vi "Stage 3.4 Placing hardware into subVIs.vi"() -> ()   [LabVIEW 2020]
uses:
  HRM-Stage3-User_events.ctl
  HRM-Stage3-init_cluster.ctl
panel:
  out "Process Error":errorcluster
  out "error out":errorcluster
  out "error out Hardware":errorcluster
  in  "Addition signal to remove (0) [s]":dbl
  out "Pulse":dbl
  out "Filtered":waveform(dbl)(graph)
  in  "Samples size (10) [s]":i32=10
  out "unfiltered wf":waveform(dbl)(graph)
  in  "Stop":bool
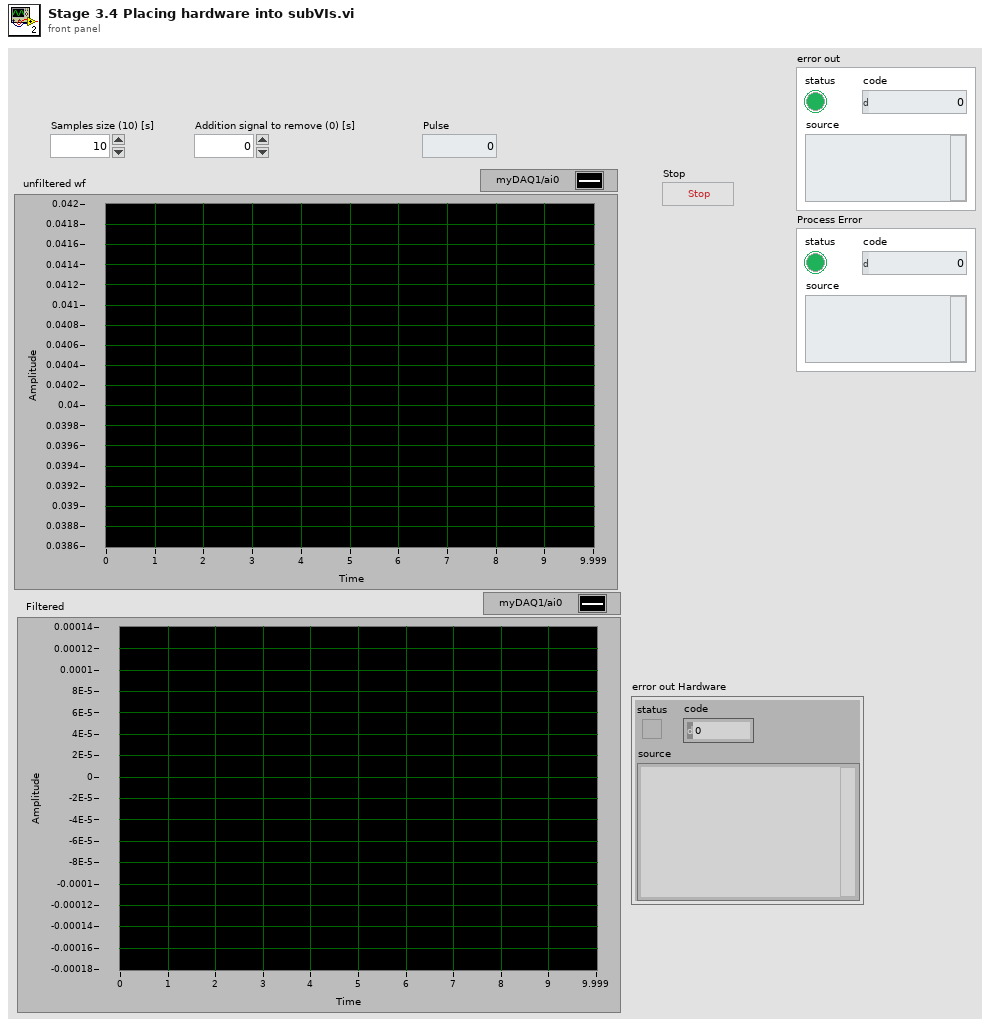
[diagram p1: front panel]
types:
  T1 = typedef "HRM-Stage3-init_cluster.ctl" = cluster{"User events":T2}
  T2 = typedef "HRM-Stage3-User_events.ctl" = cluster{"Signal to remove":refnum<user-event>, "Sample size":refnum<user-event>, "Filtered wf":refnum<user-event>, "Unfiltered wf":refnum<user-event>, "Raw wf":refnum<user-event>, "Pulse":refnum<user-event>, "Stop":refnum<user-event>, "Feedback":refnum<user-event>}
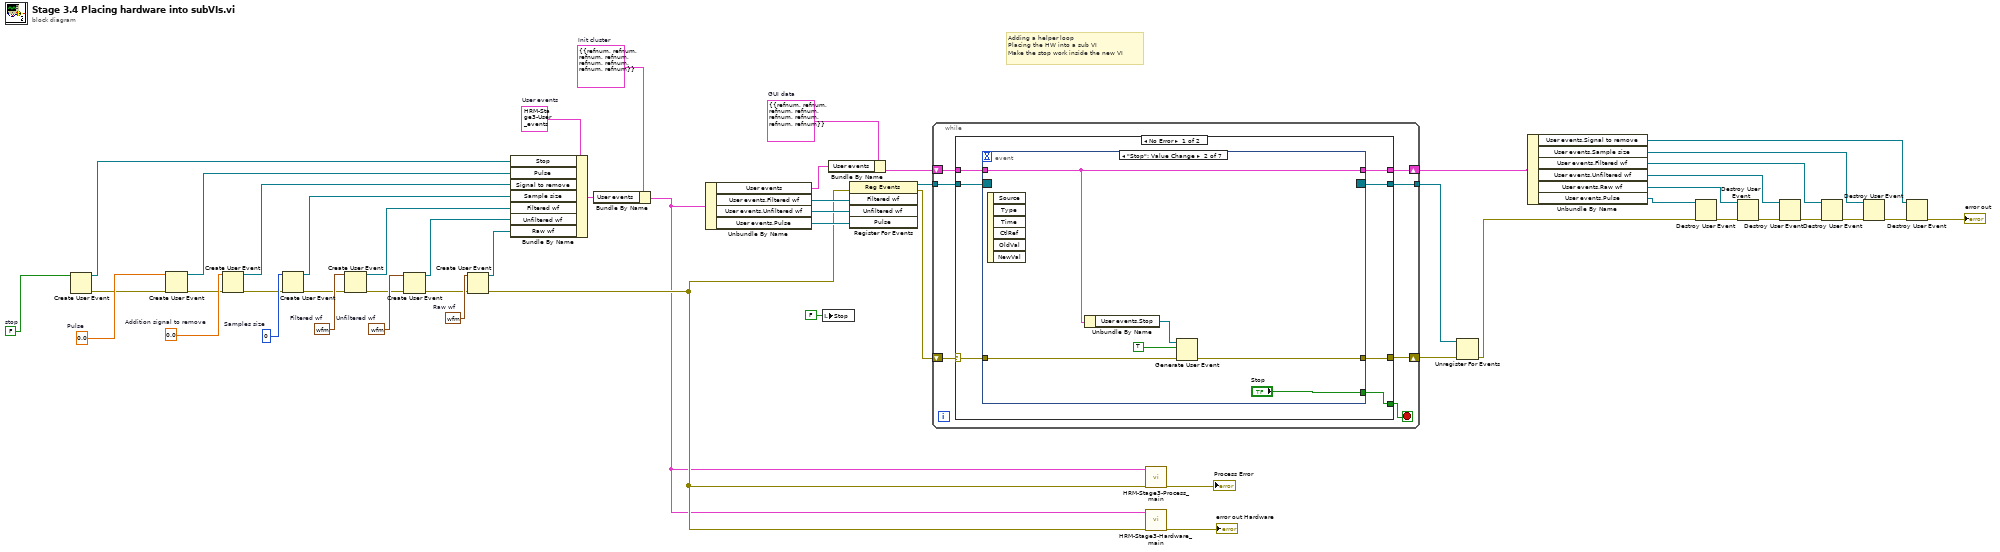
[diagram p0: block diagram]
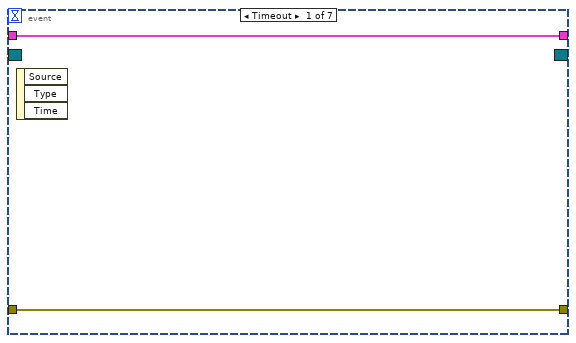
[diagram p2: hidden frame]
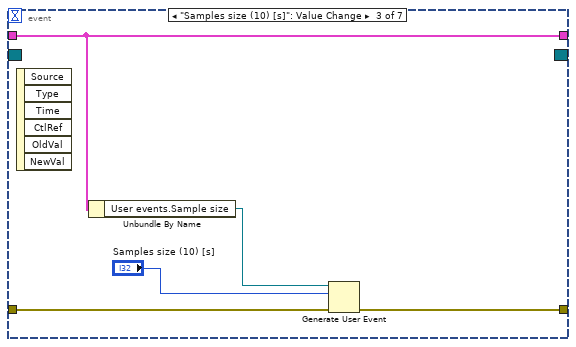
[diagram p3: hidden frame]
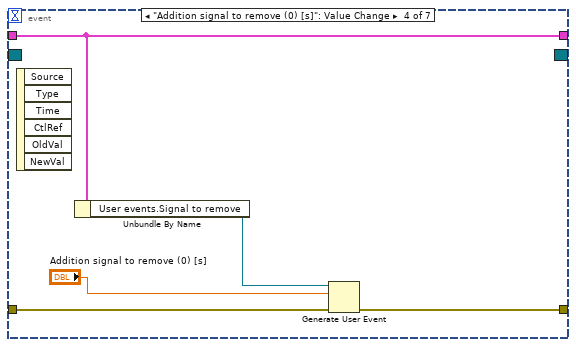
[diagram p4: hidden frame]
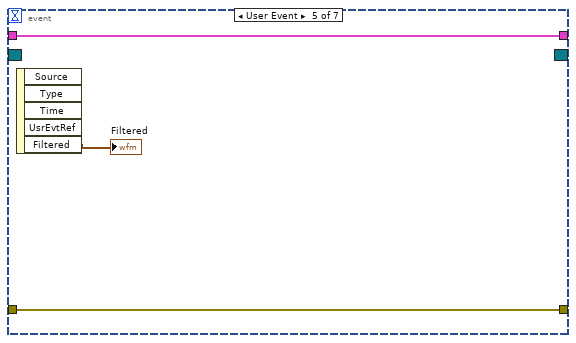
[diagram p5: hidden frame]
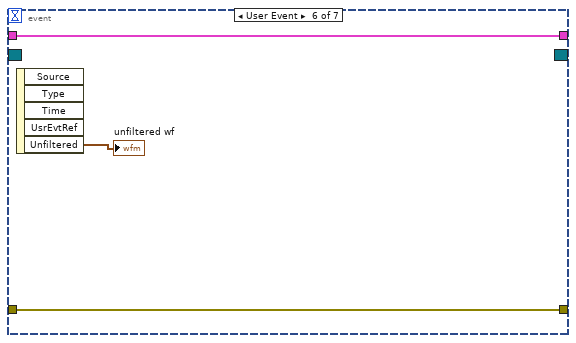
[diagram p6: hidden frame]
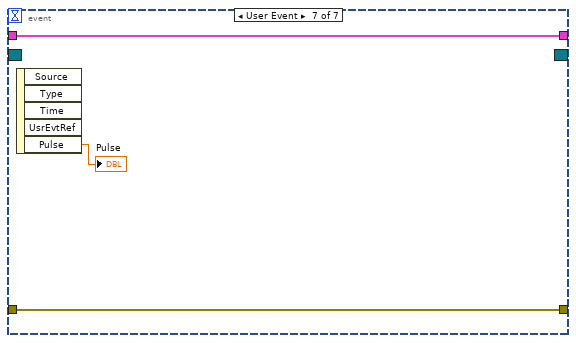
[diagram p7: hidden frame]
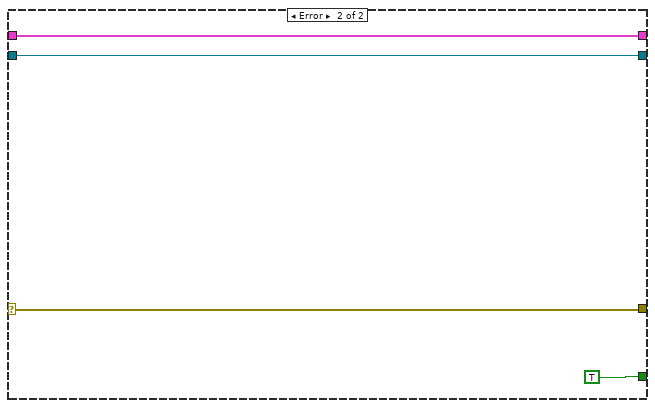
[diagram p8: hidden frame]
diagram:
  w8 = FALSE  # stop
  w14 = T1 {"User events"={"Signal to remove"=refnum, "Sample size"=refnum, "Filtered wf"=refnum, "Unfiltered wf"=refnum, "Raw wf"=refnum, "Pulse"=refnum, "Stop"=refnum, "Feedback"=refnum}}  # Init cluster
  w33 = cluster{"User events":T2} {"User events"={"Signal to remove"=refnum, "Sample size"=refnum, "Filtered wf"=refnum, "Unfiltered wf"=refnum, "Raw wf"=refnum, "Pulse"=refnum, "Stop"=refnum, "Feedback"=refnum}}  # GUI data
  w37 = 0.0  # Pulse
  w43 = T2 {"Signal to remove"=refnum, "Sample size"=refnum, "Filtered wf"=refnum, "Unfiltered wf"=refnum, "Raw wf"=refnum, "Pulse"=refnum, "Stop"=refnum, "Feedback"=refnum}  # User events
  w48 = 0  # Samples size
  w49 = 0.0  # Addition signal to remove
  w50 = waveform(dbl) {"t0"=timestamp(0 s since 1904-01-01), "dt"=1.0, "Y"=[]}  # Filtered wf
  w51 = waveform(dbl) {"t0"=timestamp(0 s since 1904-01-01), "dt"=1.0, "Y"=[]}  # Unfiltered wf
  w52 = waveform(dbl) {"t0"=timestamp(0 s since 1904-01-01), "dt"=1.0, "Y"=[]}  # Raw wf
  # "Adding a helper loop\nPlacing the HW into a sub VI\nMake the stop work inside the new VI"
  n1 = Create User Event(user event datatype=w8) -> (user event=w6:refnum<user-event>, error out=w7:errorcluster)  [unwired: 1 in]
  n2 = Create User Event(user event datatype=w37, error in=w7) -> (user event=w36:refnum<user-event>, error out=w35:errorcluster)
  n3 = Create User Event(user event datatype=w49, error in=w35) -> (user event=w42:refnum<user-event>, error out=w44:errorcluster)
  n4 = Create User Event(user event datatype=w48, error in=w44) -> (user event=w41:refnum<user-event>, error out=w45:errorcluster)
  n5 = Create User Event(user event datatype=w50, error in=w45) -> (user event=w40:refnum<user-event>, error out=w46:errorcluster)
  n6 = Create User Event(user event datatype=w51, error in=w46) -> (user event=w39:refnum<user-event>, error out=w47:errorcluster)
  n7 = Create User Event(user event datatype=w52, error in=w47) -> (user event=w38:refnum<user-event>, error out=w4:errorcluster)
  n8 = Bundle By Name(cluster=w43, "Stop"=w6, "Pulse"=w36, "Signal to remove"=w42, "Sample size"=w41, "Filtered wf"=w40, "Unfiltered wf"=w39, "Raw wf"=w38) -> (w13:T2)
  n9 = Bundle By Name(cluster=w14, "User events"=w13) -> (w3:T1)
  n10 = Unbundle By Name(w3) -> ("User events"=w12:T2, "User events.Filtered wf"=w11:refnum<user-event>, "User events.Unfiltered wf"=w10:refnum<user-event>, "User events.Pulse"=w9:refnum<user-event>)
  n11 = local write "Stop"(FALSE ("Stop")) -> ()
  n12 = Bundle By Name(cluster=w33, "User events"=w12) -> (w15:cluster{"User events":T2})
  n13 = register-events(error in=w4, w11, w10, w9) -> (reference out=w34:refnum<event-registration>, error out=w32:errorcluster)  [unwired: 1 in]
  n14 = while {
    tunnel: w34 -> [w59]
    shift-right: [w55] -> w30
    shift-left: w32 -> [w56]
    shift-right: [w54] -> w29
    shift-left: w15 -> [w58]
    tunnel: [w53] -> w31
    stop <- w57 stop-if-true
    n15 = case shown="No Error" w56 {
      selector: w56 -> [w63 w96]
      tunnel: [w64 TRUE ("Stop")] -> w57
      tunnel: [w62 w96] -> w55
      tunnel: w59 -> [w66 w94]
      tunnel: w58 -> [w65 w95]
      tunnel: [w61 w95] -> w54
      tunnel: [w60 w94] -> w53
      frame No Error {
        n16 = event shown="[1] \"Stop\": Value Change" {
          selector: w66 -> [_ _ _ _ _ _ _]
          dyn-events: [_ _ _ _ _ _ _] -> w60
          timeout: _ -> [_ _ _ _ _ _ _]
          tunnel: w65 -> [w68 w73 w77 w82 w86 w89 w92]
          tunnel: [_ "Stop" _ _ _ _ _] -> w64
          tunnel: [w67 w70 w78 w83 w87 w90 w93] -> w62
          tunnel: w63 -> [w67 w71 w79 w84 w87 w90 w93]
          tunnel: [w68 w73 w77 w82 w86 w89 w92] -> w61
          event Timeout {
            n17 = event-data() -> ()  [unwired: 1 in, 3 out]
          }
          event "Stop": Value Change {
            n18 = event-data() -> ()  [unwired: 1 in, 6 out]
            n19 = Unbundle By Name(w73) -> ("User events.Stop"=w72:refnum<user-event>)
            n20 = Generate User Event(user event=w72, event data cluster=TRUE ("event data"), error in=w71) -> (error out=w70:errorcluster)  [unwired: 1 in, 1 out]
          }
          event "Samples size (10) [s]": Value Change {
            n21 = event-data() -> ()  [unwired: 1 in, 6 out]
            n22 = Unbundle By Name(w77) -> ("User events.Sample size"=w76:refnum<user-event>)
            n23 = Generate User Event(user event=w76, event data cluster="Samples size (10) [s]", error in=w79) -> (error out=w78:errorcluster)  [unwired: 1 in, 1 out]
          }
          event "Addition signal to remove (0) [s]": Value Change {
            n24 = event-data() -> ()  [unwired: 1 in, 6 out]
            n25 = Unbundle By Name(w82) -> ("User events.Signal to remove"=w81:refnum<user-event>)
            n26 = Generate User Event(user event=w81, event data cluster="Addition signal to remove (0) [s]", error in=w84) -> (error out=w83:errorcluster)  [unwired: 1 in, 1 out]
          }
          event User Event {
            n27 = event-data() -> ("Filtered"=→"Filtered":waveform(dbl))  [unwired: 1 in, 4 out]
          }
          event User Event {
            n28 = event-data() -> ("Unfiltered"=→"unfiltered wf":waveform(dbl))  [unwired: 1 in, 4 out]
          }
          event User Event {
            n29 = event-data() -> ("Pulse"=→"Pulse":dbl)  [unwired: 1 in, 4 out]
          }
        }
      }
      frame Error {
      }
    }
  }
  n30 = call "HRM-Stage3-Process_main.vi"("error in (no error)"=w4, "Init cluster"=w3) -> ("error out"=→"Process Error":errorcluster)  [unwired: 9 in]
  n31 = call "HRM-Stage3-Hardware_main.vi"("error in (no error)"=w4, "Init cluster"=w3) -> ("error out"=→"error out Hardware":errorcluster)  [unwired: 9 in]
  n32 = Unregister For Events(event registration refnum=w31, error in=w30) -> (error out=w17:errorcluster)
  n33 = Unbundle By Name(w29) -> ("User events.Signal to remove"=w18:refnum<user-event>, "User events.Sample size"=w19:refnum<user-event>, "User events.Filtered wf"=w20:refnum<user-event>, "User events.Unfiltered wf"=w21:refnum<user-event>, "User events.Raw wf"=w22:refnum<user-event>, "User events.Pulse"=w23:refnum<user-event>)
  n34 = Destroy User Event(user event=w23, error in=w17) -> (error out=w24:errorcluster)
  n35 = Destroy User Event(user event=w22, error in=w24) -> (error out=w28:errorcluster)
  n36 = Destroy User Event(user event=w21, error in=w28) -> (error out=w27:errorcluster)
  n37 = Destroy User Event(user event=w20, error in=w27) -> (error out=w26:errorcluster)
  n38 = Destroy User Event(user event=w19, error in=w26) -> (error out=w25:errorcluster)
  n39 = Destroy User Event(user event=w18, error in=w25) -> (error out=→"error out":errorcluster)
